vi "QX_PrepareDAQ.vi"(8 "Error in":errorcluster, 9 "BufferTimeout":i32=3000, 11 "DevRef[]":T1(array[cluster])) -> (0 "Error out":errorcluster, 2 "DaqMeasurement":refnum<k24>)   [LabVIEW 2016]
doc: "Prepares a continuous measurement.\nIf any signal does not belong to the given devices or the device does not support the demanded sample rate, an error will be thrown.\n\nDevicesAndSignals: Array of devices and their signals that have been chosen for measurement\nDaqMeasurement: Reference to the DaqMearurement object that handles the measurement\nBufferTimeout: Buffer timeout in milliseconds (default is 3000ms). Used to calculate size of internal circular buffer. At least there is a buffer of 1000 values for each signal. Normally the buffer size is (bufferTimeout/1000)*sample rate of the signal, prior added to the measurement (E.g.: Signal.SampleRate=1200Hz, bufferTimeOut=1000ms => size of internal circular buffer is 1200 entries)"
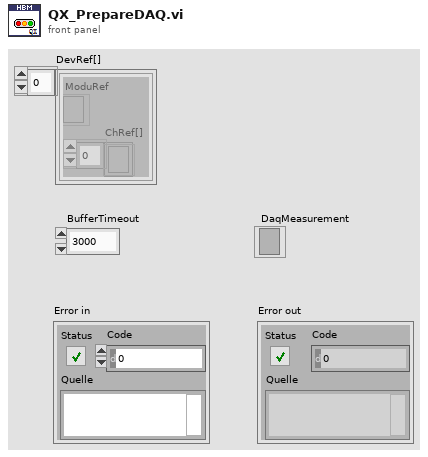
[diagram p1: front panel]
types:
  T1 = cluster{"ModuRef":refnum<k24>, "ChRef[]":refnum<k24>[]}[]
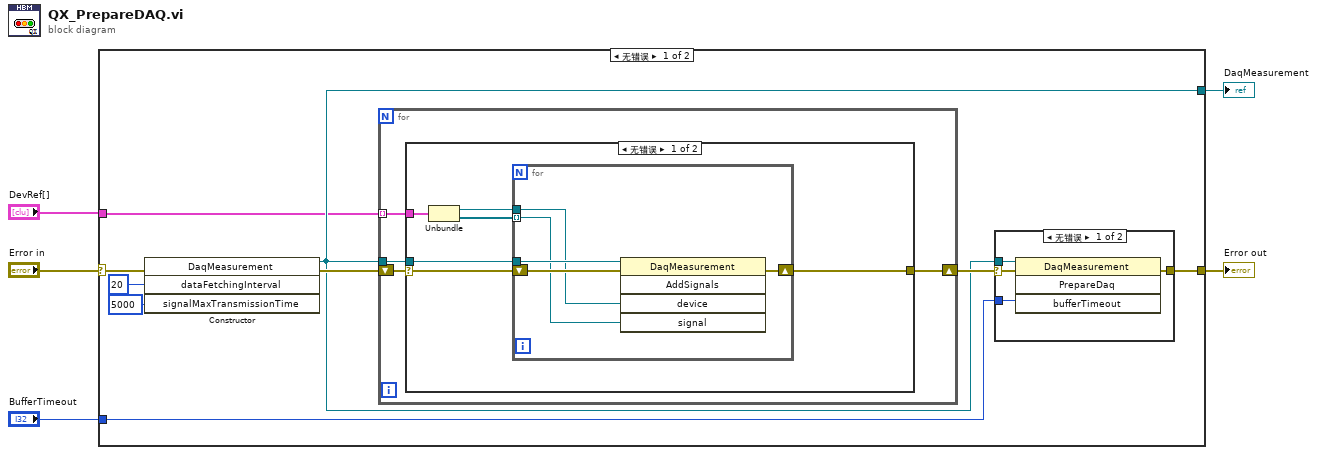
[diagram p0: block diagram]
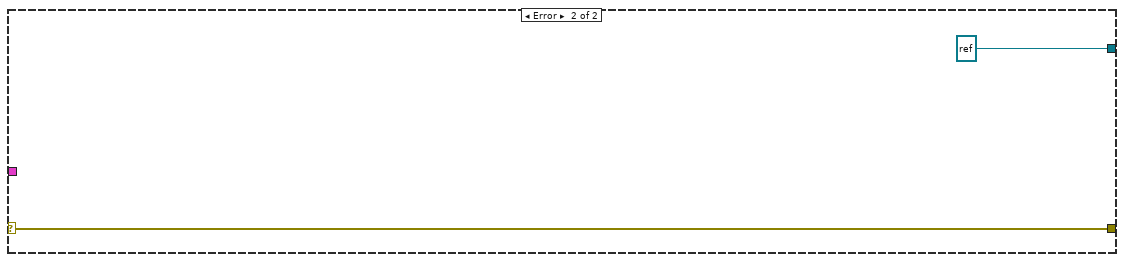
[diagram p4: hidden frame]
diagram:
  n1 = case shown="无错误" "Error in" {
    selector: "Error in" -> [w13 w37]
    tunnel: [w10 w37] -> w5
    tunnel: [w9 refnum<k24> refnum ("new reference")] -> w3
    tunnel: "DevRef[]" -> [w6 _]
    tunnel: "BufferTimeout" -> [w8 _]
    frame No Error {
      n2 = constructor class="DaqMeasurement"(error in=w13, "dataFetchingInterval"=20, "signalMaxTransmissionTime"=5000) -> (reference out=w9:refnum<k24>, error out=w12:errorcluster)  [unwired: 2 in, 3 out]
      n3 = for {
        tunnel: w9 -> [w23]
        shift-right: [w22] -> w11
        shift-left: w12 -> [w21]
        tunnel: w6 -> [w20] mode=indexing
        n4 = case shown="无错误" w21 {
          selector: w21 -> [w27 w35]
          tunnel: w23 -> [w29 _]
          tunnel: [w28 w35] -> w22
          tunnel: w20 -> [w26 _]
          frame No Error {
            n5 = Unbundle(w26) -> ("ModuRef"=w25:refnum<k24>, "ChRef[]"=w24:refnum<k24>[])
            n6 = for {
              tunnel: w29 -> [w34]
              shift-right: [w33] -> w28
              shift-left: w27 -> [w32]
              tunnel: w25 -> [w30]
              tunnel: w24 -> [w31] mode=indexing
              n7 = invoke on="Methodenknoten" class="DaqMeasurement" method="AddSignals"(reference=w34, error in=w32, "device"=w30, "signal"=w31) -> (error out=w33:errorcluster)  [unwired: 1 in, 4 out]
            }
          }
          frame Error {
          }
        }
      }
      n8 = case shown="无错误" w11 {
        selector: w11 -> [w17 w19]
        tunnel: [w16 w19] -> w10
        tunnel: w9 -> [w18 _]
        tunnel: w8 -> [w15 _]
        frame No Error {
          n9 = invoke on="Methodenknoten" class="DaqMeasurement" method="PrepareDaq"(reference=w18, error in=w17, "bufferTimeout"=w15) -> (error out=w16:errorcluster)  [unwired: 1 in, 3 out]
        }
        frame Error {
        }
      }
    }
    frame Error {
    }
  }
  "Error out" <- w5
  "DaqMeasurement" <- w3
